vi "Configure.vi"(8 "error in (no error)":errorcluster, 9 "DAQ Parameters":T1={"Points Per A-Scan"=1024, "A-Scans Per B-Scan"=250, "Number of B-Scans"=1, "A-Scans Per Transfer"=1, "Trigger Voltage"=0.0, "Trigger Source"=enum."External", "Trigger Slope"=enum."Rising", "Channel"=enum."Channel 1", "Clock"=enum."Internal Clock", "Bits per Sample"=0.0, "Range"=0.0}, 10 "Scanning":T6={"Fast Axis Offset"=10.0, "Slow Axis Offset"=0.0, "Slow Axis Amp"=20.0, "Fast Axis Amp"=20.0, "Scan Pattern"=enum."Raster"} {"Fast Axis Amp" max=20 format="%#.2f"; "Slow Axis Amp" max=20 format="%#.2f"; "Slow Axis Offset" max=10 format="%#.2f"; "Fast Axis Offset" max=10 format="%#.2f"}, 11 "Galvo in":refnum<class "Galvo.lvclass">) -> (0 "error out":errorcluster, 3 "Galvo out":refnum<class "Galvo.lvclass">)   [LabVIEW 2014, in "Galvo.lvclass"]
uses:
  Galvo.lvclass
  Scanning Cluster.ctl
  DAQ/DAQ Parameters.ctl
  DAQ/Trigger Source.ctl
  DAQ/Trigger Slope.ctl
  Type Defs/OCT DAQ Channel Data Type.ctl
  DAQ/Clock Control.ctl
  Galvo.lvclass/Galvo.ctl
  DAQ/DAQ Class.lvclass
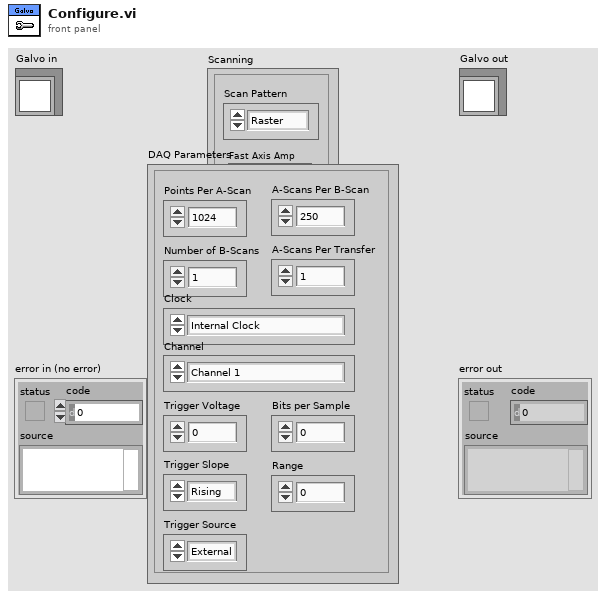
[diagram p1: front panel]
types:
  T1 = typedef "DAQ Class.lvclass/DAQ Parameters.ctl" = cluster{"Points Per A-Scan":u32, "A-Scans Per B-Scan":u32, "Number of B-Scans":u32, "A-Scans Per Transfer":u32, "Trigger Voltage":sgl, "Trigger Source":T2, "Trigger Slope":T3, "Channel":T4, "Clock":T5, "Bits per Sample":dbl, "Range":dbl}
  T2 = typedef "DAQ Class.lvclass/Trigger Source.ctl" = enum16{"External", "Channel A", "Channel B"}
  T3 = typedef "DAQ Class.lvclass/Trigger Slope.ctl" = enum16{"Rising", "Falling"}
  T4 = typedef "OCT DAQ Channel Data Type.ctl" = enum16{"Channel 1", "Channel 2", "Channel 1 and 2"}
  T5 = typedef "DAQ Class.lvclass/Clock Control.ctl" = enum16{"Internal Clock", "External Clock"}
  T6 = typedef "Galvo.lvclass/Scanning Cluster.ctl" = cluster{"Fast Axis Offset":sgl, "Slow Axis Offset":sgl, "Slow Axis Amp":sgl, "Fast Axis Amp":sgl, "Scan Pattern":enum16{"Raster"}}
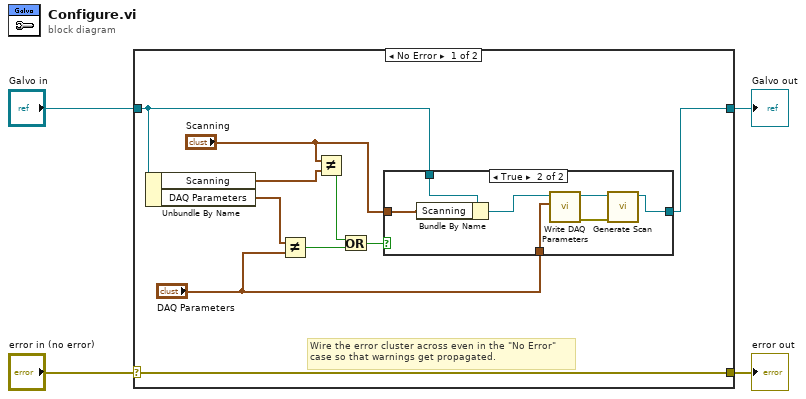
[diagram p0: block diagram]
diagram:
  n1 = case shown="No Error" "error in (no error)" {
    selector: "error in (no error)" -> [w14 w24]
    tunnel: [w14 w24] -> w3
    tunnel: [w6 w23] -> w1
    tunnel: "Galvo in" -> [w12 w23]
    frame No Error {
      # "Wire the error cluster across even in the \"No Error\"\ncase so that warnings get propagated."
      n2 = Unbundle By Name(w12) -> ("Scanning"=w11:T6, "DAQ Parameters"=w8:T1)
      n3 = Not Equal?(x=w8, y="DAQ Parameters") -> (x != y?=w7:bool)
      n4 = Not Equal?(x="Scanning", y=w11) -> (x != y?=w9:bool)
      n5 = Or(x=w9, y=w7) -> (x .or. y?=w10:bool)
      n6 = case shown="True" w10 {
        tunnel: "Scanning" -> [_ w22]
        tunnel: w12 -> [w15 w20]
        tunnel: [w15 w17] -> w6
        tunnel: "DAQ Parameters" -> [_ w21]
        frame False {
        }
        frame True {
          n7 = Bundle By Name(cluster=w20, "Scanning"=w22) -> (w16:refnum<class "Galvo.lvclass">)
          n8 = call-dynamic "Write DAQ Parameters.vi"("DAQ Parameters"=w21, "Galvo in"=w16) -> ("error out"=w18:errorcluster, "Galvo out"=w19:refnum<class "Galvo.lvclass">)  [unwired: 8 in]
          n9 = call-dynamic "Generate Scan.vi"("error in (no error)"=w18, "Galvo in"=w19) -> ("Galvo out"=w17:refnum<class "Galvo.lvclass">)  [unwired: 8 in, 1 out]
        }
      }
    }
    frame Error {
    }
  }
  "error out" <- w3
  "Galvo out" <- w1
